vi "MenuSlider.vi"(7 "State":enum16{"Reset", "Slide"}(ring), 8 "Error In":errorcluster, 9 "Open Position":u32, 10 "Close Position":u32, 11 "Splitter Refnum":refnum<vi>) -> (0 "Error Out":errorcluster)   [LabVIEW 2009]
doc: "Takes a reference to a Splitter bar and slides between the Open and Closed position. The VI must be set to Reentrant if multiple Splitter bars are used."
uses:
  <vilib>/Analysis/NI_AALBase.lvlib
  <vilib>/Analysis/1siggen.llb/Ramp Pattern by Samples.vi
panel:
  # "Input"
  # "Output"
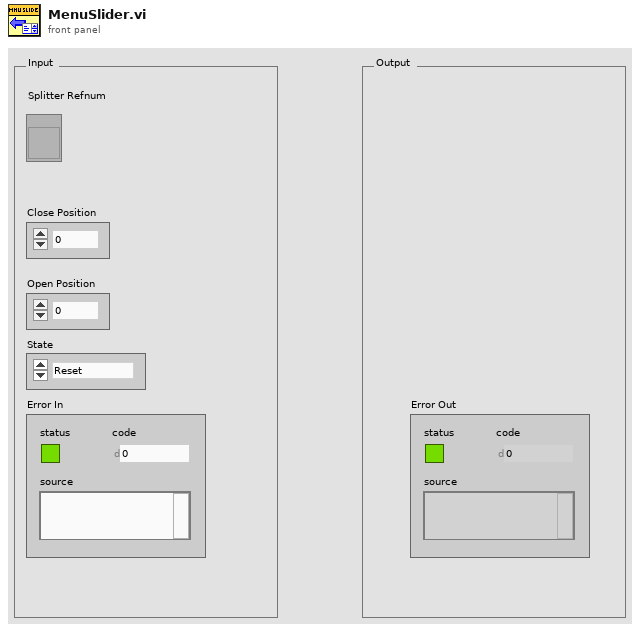
[diagram p1: front panel]
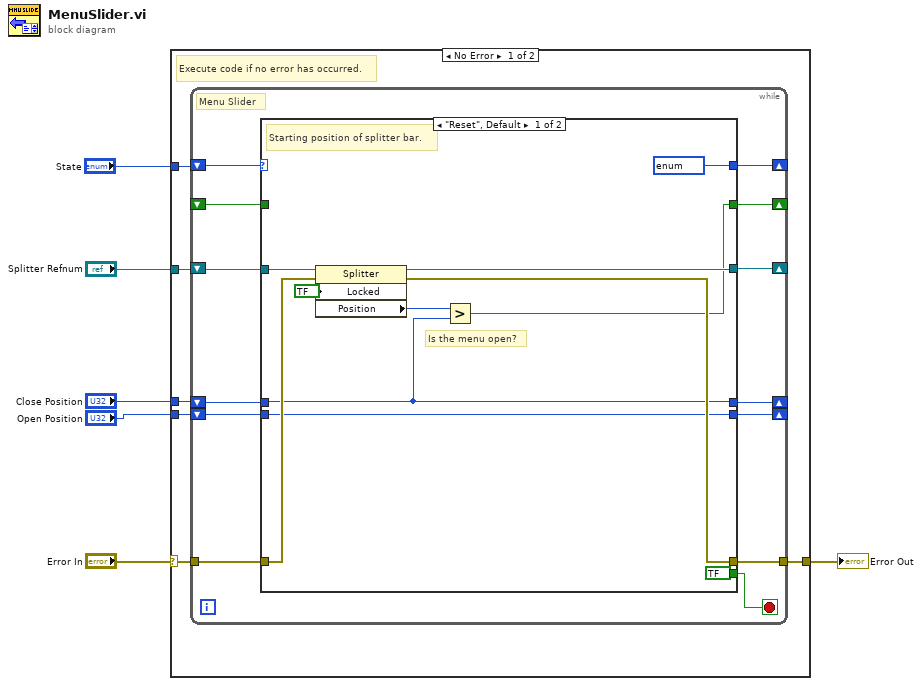
[diagram p0: block diagram]
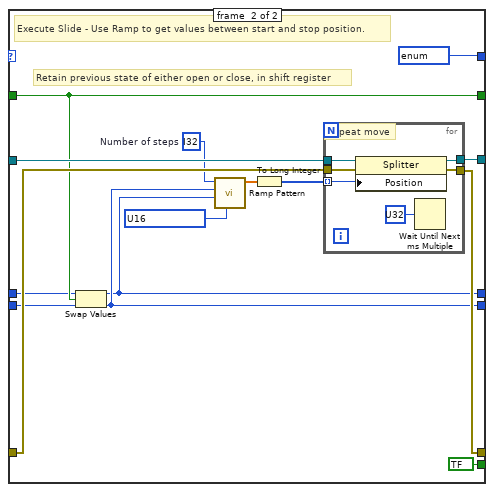
[diagram p2: hidden frame]
diagram:
  n1 = case shown="No Error" "Error In" {
    selector: "Error In" -> [w11 w58]
    tunnel: [w10 w58] -> w5
    tunnel: "Splitter Refnum" -> [w12 _]
    tunnel: "State" -> [w9 _]
    tunnel: "Close Position" -> [w8 _]
    tunnel: "Open Position" -> [w7 _]
    frame #0 {
      # "Execute code if no error has occurred."
      n2 = while {
        tunnel: w11 -> [w23]
        shift-right: [w24] -> _
        shift-left: w12 -> [w25]
        tunnel: [w22] -> w10
        shift-right: [w19] -> _
        shift-left: _ -> [w18]
        shift-right: [w15] -> _
        shift-left: w7 -> [w20]
        shift-right: [w16] -> _
        shift-left: w8 -> [w21]
        shift-right: [w13] -> _
        shift-left: w9 -> [w17]
        stop <- w14 stop-if-true
        # "Menu Slider"
        n3 = case shown="\"Reset\", Default" w17 {
          tunnel: w25 -> [w36 w51]
          tunnel: [w35 w49] -> w24
          tunnel: w23 -> [w34 w47]
          tunnel: [w33 w46] -> w22
          tunnel: w21 -> [w27 w40]
          tunnel: w20 -> [w26 w39]
          tunnel: [w28 w45] -> w19
          tunnel: w18 -> [_ w45]
          tunnel: [w27 w37] -> w16
          tunnel: [w26 w38] -> w15
          tunnel: [bool ? bool ?] -> w14
          tunnel: [enum16{"Reset", "Slide"} ? ("State") enum16{"Reset", "Slide"} ? ("State")] -> w13
          frame #0 {
            # "Is the menu open?"
            # "Starting position of splitter bar."
            n4 = property class="Splitter"(reference=w36, error in=w34, "Locked"=bool ? ("Splitter Position Locked")) -> (reference out=w35:refnum<vi>, error out=w33:errorcluster, "Position"=w29:i32)
            n5 = Greater?(x=w29, y=w27) -> (0:w28:bool)
          }
          frame #1 {
            w44 = i32 ?  # Number of steps
            w50 = u16 ? items=["Linear", "Logarithmic"] ("type")
            # "Retain previous state of either open or close, in shift register"
            # "Execute Slide - Use Ramp to get values between start and stop position."
            n6 = Swap Values(12:w40, 13:w45, 14:w39) -> (1:w37:u32, 3:w38:u32)
            n7 = call-poly <vilib>:"Ramp Pattern.vi"("type"=w50, "start"=w37, "end"=w38, "samples"=w44) -> ("Ramp Pattern"=w48:dbl[])  [unwired: 6 in, 1 out]
            n8 = To Long Integer(number=w48) -> (32bit integer=w43:i32[])
            n9 = for {
              tunnel: w51 -> [w57]
              tunnel: w47 -> [w56]
              tunnel: [w55] -> w46
              tunnel: [w54] -> w49
              tunnel: w43 -> [w52] mode=indexing
              # "Repeat move"
              n10 = property class="Splitter"(reference=w57, error in=w56, "Position"=w52) -> (reference out=w54:refnum<vi>, error out=w55:errorcluster)
              n11 = Wait Until Next ms Multiple(millisecond multiple=u32 ?) -> ()  [unwired: 1 out]
            }
          }
        }
      }
    }
    frame #1 {
    }
  }
  "Error Out" <- w5
